vi "coin.vi"(0 "Image In":T2, 7 "error in":errorcluster) -> (20 "Image Out":T2, 21 "Circles (Shape Detection 1)":T1(array[cluster]) {"Position"."Y" format="%.2f"; "Position"."X" format="%.2f"}, 22 "Number of Matches (Shape Detection 1)":i32, 27 "error out":errorcluster)   [LabVIEW 2018]
uses:
  <vilib>/vision/Image Controls.llb/IMAQ Image.ctl
  <vilib>/vision/NI_Vision_Development_Module.lvlib
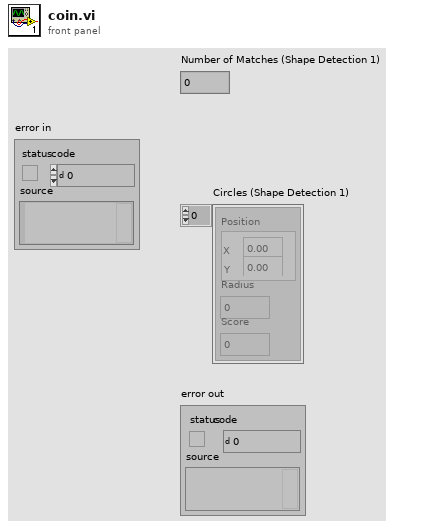
[diagram p1: front panel]
types:
  T1 = cluster{"Position":cluster{"X":sgl, "Y":sgl}, "Radius":dbl, "Score":dbl}[]
  T2 = typedef "IMAQ Image.ctl" = refnum<image>
  T3 = cluster{"Extraction Mode":u32, "Edge Threshold":i32, "Edge Filter Size":u32, "Min Length":i32, "Row Search Step Size":i32, "Col Search Step Size":i32, "Max Endpoint Gap":i32, "Closed":bool, "Subpixel":bool}
  T4 = cluster{"Rotation":bool, "Scale":bool, "Occlusion":bool, "Range Settings":cluster{"Match Constraints":u32, "Min":dbl, "Max":dbl}[]}
  T5 = cluster{"Global Rectangle":i32[], "Contours":cluster{"ID":enum32{"External", "Internal"}, "Type":u32, "Coordinates":i32[]}[]}
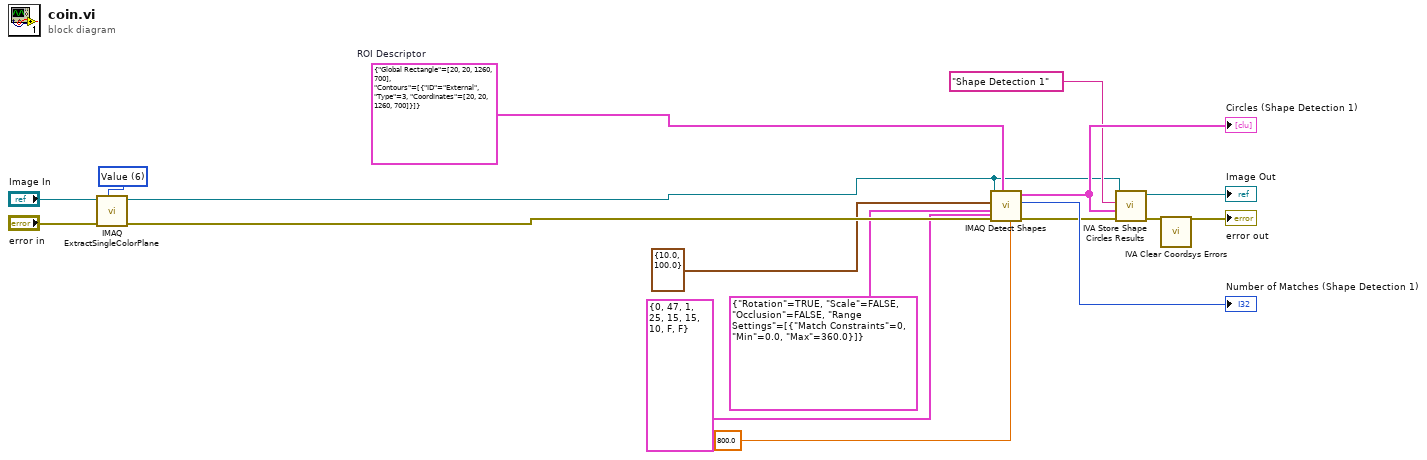
[diagram p0: block diagram]
diagram:
  w8 = T5 {"Global Rectangle"=[20, 20, 1260, 700], "Contours"=[{"ID"=enum."External", "Type"=3, "Coordinates"=[20, 20, 1260, 700]}]}  # ROI Descriptor
  w17 = 6 items=["Red", "Green", "Blue", "Hue", "Saturation", "Luminance", "Value", "Intensity"] ("Color Plane")
  n1 = call "IMAQ ExtractSingleColorPlane"("Color Plane"=w17, "error in (no error)"="error in", "Image Src"="Image In") -> ("error out"=w14:errorcluster, "Image Dst Out"=w3:T2)  [unwired: 1 in, 6 out]
  n2 = call-poly "IMAQ Detect Shapes"("Minimum match score"=800.0, "Curve Parameters"=T3 {"Extraction Mode"=0, "Edge Threshold"=47, "Edge Filter Size"=1, "Min Length"=25, "Row Search Step Size"=15, "Col Search Step Size"=15, "Max Endpoint Gap"=10, "Closed"=FALSE, "Subpixel"=FALSE}, "ROI Descriptor"=w8, "error in (no error)"=w14, "Match Options"=T4 {"Rotation"=TRUE, "Scale"=FALSE, "Occlusion"=FALSE, "Range Settings"=[{"Match Constraints"=0, "Min"=0.0, "Max"=360.0}]}, "Circle Descriptor"=cluster{"Min Radius":dbl, "Max Radius":dbl} {"Min Radius"=10.0, "Max Radius"=100.0}, "Image"=w3) -> ("error out"=w5:errorcluster, "Number of Matches Returned"=→"Number of Matches (Shape Detection 1)":i32, "Circles"=w7:T1)  [unwired: 2 out]
  "Circles (Shape Detection 1)" <- w7
  n3 = call <vilib>:"IVA Store Shape Circles Results.vi"("error in (no error)"=w5, "Circles"=w7, "Step Name"="Shape Detection 1", "Image in"=w3) -> ("error out"=w2:errorcluster, "Image dup"=→"Image Out":T2)  [unwired: 6 out]
  n4 = call <vilib>:"IVA Clear Coordsys Errors.vi"("error in (no error)"=w2) -> ("error out"=→"error out":errorcluster)  [unwired: 10 in]
